vi "SigSyn (G3)-Create (1D).vi"(0 "StimChans In":T1[](array[typedef]) {"Filter"."Stages"."IIR Filter"."Forward Coefficients" format="%.4f"; "Filter"."Stages"."IIR Filter"."Reverse Coefficients" format="%.4f"}, 1 "Apply multipliers? (F)":bool, 5 "Sampling Rate (Hz)":dbl=100000.0, 7 "Npts":i32=500, 9 "Rep Num":i32=-1, 11 "error in (no error)":errorcluster, 12 "Zero unused (F)":bool) -> (4 "StimChans Out":T1[](array[typedef]) {"Filter"."Stages"."IIR Filter"."Forward Coefficients" format="%.4f"; "Filter"."Stages"."IIR Filter"."Reverse Coefficients" format="%.4f"}, 6 "Waveform":dbl[][](array[numeric]), 8 "Multipliers":dbl[](array[numeric]), 15 "error out":errorcluster)   [LabVIEW 2020]
uses:
  XControls/Stimulus Channel (G3)/Full Stimulus Channel Data.ctl
  XControls/Waveform XControls/Waveform (G3)/Waveform Data.ctl
  Waveform VIs/Waveform Enum (V3).ctl
  XControls/Waveform XControls/Tone (G3)/Tone.Properties.ctl
  Waveform VIs/Pulse Train VIs/Pulse Train Params.ctl
  Waveform VIs/Pulse Train VIs/Pulse Polarity.ctl
  Waveform VIs/Pulse Train VIs/PT-Continuous State.ctl
  Waveform VIs/Noise VIs/Noise (G3).ctl
  Waveform VIs/Noise VIs/Noise (G3).Properties.ctl
  Waveform VIs/Noise VIs/Noise (G3).Data.ctl
  Waveform VIs/File VIs/StimFile-Params.ctl
  Waveform VIs/FM Sweep VIs/FM Sweep Params.ctl
  Waveform VIs/Chirp Train VIs/Chirp Train.ctl
  Waveform VIs/Chirp Train VIs/Chirp Train Params.ctl
  Waveform VIs/Complex Tone VIs/CT-Params.ctl
  Waveform VIs/Complex Tone VIs/CT-Phase Enum.ctl
  Waveform VIs/Complex Tone VIs/CT-Runtime Data.ctl
  XControls/Waveform XControls/FM Tone/Data.ctl
  XControls/Waveform XControls/Vowel/Vowel.Properties.ctl
  Waveform VIs/Ramp VIs/Ramp.Properties.ctl
  XControls/Filter (G3)/Filter Data.ctl
  XControls/Filter (G3)/Filter Type.ctl
  Filter VIs/Filter-Bandwidth Units.ctl
  Controls/Burst XCtl/Burst Data.ctl
  XControls/Level (G3)/Level Data.ctl
  XControls/Level (G3)/Level Units (G3).ctl
  XControls/Advanced Options (G3)/Advanced Options (G3).ctl
  Modulation VIs/SAM VIs/SAM Params.ctl
  Typedefs/Destination.ctl
  PXI DAQ VIs/DAQ Engine VIs/AO Gain and Multiplier VIs/PXI Multipliers to AO Gains (1D).vi
  XControls/Filter (G3)/Filter (G3).xctl
  XControls/Level (G3)/Level (G3).xctl
  Controls/Burst XCtl/Burst Control.xctl
  XControls/Waveform XControls/Waveform (G3)/Waveform (G3).xctl
  XControls/Stimulus Channel (G3)/Stimulus Channel (G3).xctl
  XControls/Advanced Options (G3)/Advanced Options (G3).xctl
  XControls/Waveform XControls/Tone (G3)/Tone (G3).xctl
  XControls/Waveform XControls/FM Tone/FM Tone.xctl
  XControls/Waveform XControls/Vowel/Vowel.xctl
panel:
  out "Ceilings":dbl[](array[numeric])
  out "Gains":dbl[](array[numeric])
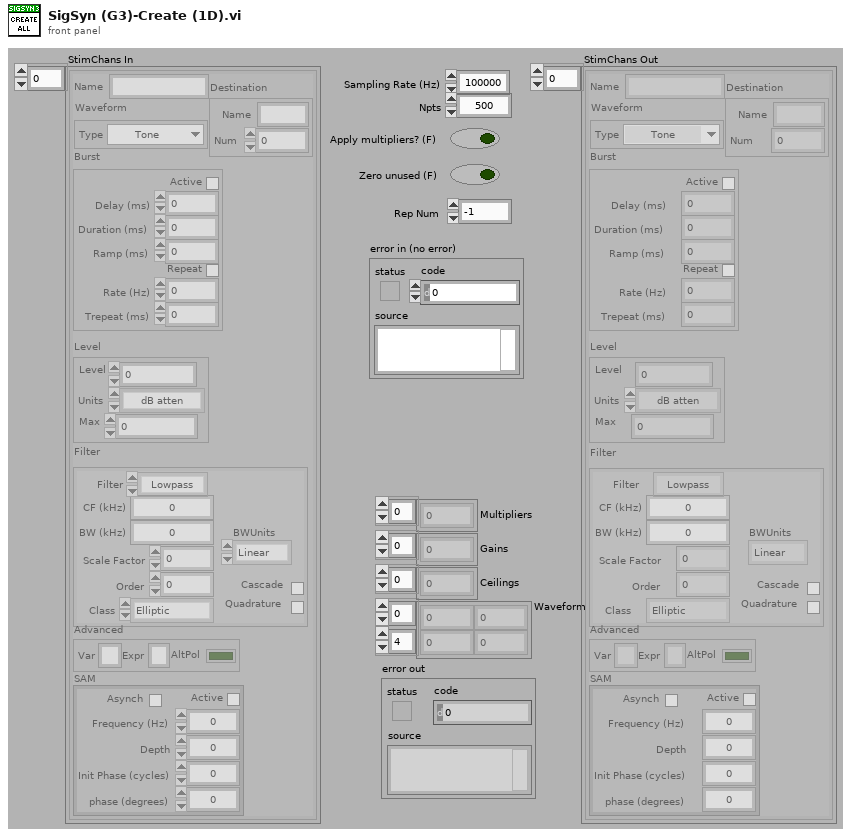
[diagram p1: front panel]
types:
  T1 = typedef "Stimulus Channel (G3).xctl/Full Stimulus Channel Data.ctl" = cluster{"Waveform":T2, "Filter":T21, "Burst":T24, "Level":T25, "Name":string, "Advanced":T27, "SAM":T28, "Destination":T29}
  T2 = typedef "Waveform (G3).xctl/Waveform Data.ctl" = cluster{"Type":T3, "Tone":T4, "Pulse Train":T5, "Noise":T8, "File":T11, "FMSweep":T12, "Chirp Train":T13, "Complex Tone":cluster{"Params":T15, "Data":T17}, "FM":T18, "Vowel":T19, "Ramp":T20}
  T3 = typedef "Waveform Enum (V3).ctl" = enum16{"OFF", "Tone", "Noise", "Pulse Train", "File", "FM Sweep", "Chirp Train", "Complex Tone", "FM Tone", "Vowel", "Ramp"}
  T4 = typedef "Tone (G3).xctl/Tone.Properties.ctl" = cluster{"Frequency (kHz)":dbl, "Phase (cycles)":dbl, "Random phase":bool}
  T5 = typedef "Pulse Train Params.ctl" = cluster{"Pulse width (us)":dbl, "Pulse rate (Hz)":dbl, "Gap (ms)":dbl, "Polarity":T6, "PT State":T7, "Asynch":bool}
  T6 = typedef "Pulse Polarity.ctl" = enum16{"POS", "NEG", "POS-NEG", "NEG-POS"}
  T7 = typedef "PT-Continuous State.ctl" = cluster{"Template":dbl[], "Nperiod":i32, "Index":i32, "Pulse Rate (Hz)":dbl, "Phase (cycles)":dbl, "Noff":i32}
  T8 = typedef "Noise (G3).ctl" = cluster{"Properties":T9, "Data":T10}
  T9 = typedef "Noise (G3).Properties.ctl" = cluster{"InvFilt":bool, "Aweight":bool, "Seed":i32, "Tokens":i32, "Brickwall":bool}
  T10 = typedef "Noise (G3).Data.ctl" = cluster{"TokenNum":i32}
  T11 = typedef "StimFile-Params.ctl" = cluster{"Filename":path, "Signal":dbl[], "Channel":i32, "stream":bool, "offset":i32, "nreps":i32, "loops":i32, "Randomize":bool, "order":i32[], "Seed":i32, "Tokens":i32}
  T12 = typedef "FM Sweep Params.ctl" = cluster{"Rate (oct/s)":dbl, "Fmin (Hz)":dbl, "Fmax (Hz)":dbl, "Ramp (ms)":dbl, "Linear":bool}
  T13 = typedef "Chirp Train.ctl" = cluster{"Params":T14, "Data":cluster{"WF":dbl[]}}
  T14 = typedef "Chirp Train Params.ctl" = cluster{"Fmin (kHz)":dbl, "Fmax (kHz)":dbl, "Compensate":bool, "Duration (ms)":dbl}
  T15 = typedef "CT-Params.ctl" = cluster{"F0 (Hz)":dbl, "Band":cluster{"Flow (Hz)":dbl, "Fhigh (Hz)":dbl}, "Phase":T16, "Min F0 (Hz)":dbl, "Max F0 (Hz)":dbl, "ContinRandPhase":bool, "Max peak factor":dbl, "Max mod depth":dbl, "MinHarmNum":i32, "MaxHarmNum":i32, "Level Mode":enum16{"per component", "overall rms"}, "% jitter":dbl}
  T16 = typedef "CT-Phase Enum.ctl" = enum16{"Cosine", "Random", "Alternating"}
  T17 = typedef "CT-Runtime Data.ctl" = cluster{"Ncomp":i32, "MinHarm":i32, "Phase":dbl[], "Amplitude":dbl[], "Npts/frame":i32, "Last F0":dbl, "Fmin":dbl, "Fmax":dbl, "Lslope":dbl, "randphase":bool, "overall rms":bool, "fmult":dbl[], "jittered":bool}
  T18 = typedef "FM Tone.xctl/Data.ctl" = cluster{"Carrier (kHz)":dbl, "ModRate (Hz)":dbl, "Depth (Hz)":dbl, "Phase (cycles)":dbl}
  T19 = typedef "Vowel.xctl/Vowel.Properties.ctl" = cluster{"Freqs":string, "Set level":enum16{"Total", "Per component"}, "Freq":dbl[], "weights":dbl[]}
  T20 = typedef "Ramp.Properties.ctl" = cluster{"Duration (ms)":dbl}
  T21 = typedef "Filter (G3).xctl/Filter Data.ctl" = cluster{"Type":T22, "CF (kHz)":dbl, "BW (kHz)":dbl, "Cascade":bool, "Quadrature":bool, "Scale Factor":dbl, "Stages":cluster{"IIR Filter":cluster{"filter structure":enum32{"IIR 2nd Order", "IIR 4th Order"}, "Reverse Coefficients":dbl[], "Forward Coefficients":dbl[]}, "State":dbl[]}[], "Class":enum16{"Elliptic", "Butterworth"}, "Order":i32, "BWUnits":T23}
  T22 = typedef "Filter (G3).xctl/Filter Type.ctl" = enum16{"OFF", "Lowpass", "Highpass", "Bandpass", "Bandstop"}
  T23 = typedef "Filter-Bandwidth Units.ctl" = enum16{"Linear", "Octaves", "Min-Max"}
  T24 = typedef "Burst Control.xctl/Burst Data.ctl" = cluster{"Active":bool, "Delay (ms)":dbl, "Duration (ms)":dbl, "Ramp (ms)":dbl, "Rate (Hz)":dbl, "Trepeat (ms)":dbl, "Repeat":bool}
  T25 = typedef "Level (G3).xctl/Level Data.ctl" = cluster{"Level":dbl, "Units":T26, "Max":dbl, "Data":cluster{"Multiplier":dbl, "Cal File":path, "Cal":cluster{"Freq (Hz)":dbl[], "Mag (dB SPL)":dbl[], "Phase (deg)":dbl[]}, "audiogram":path}}
  T26 = typedef "Level (G3).xctl/Level Units (G3).ctl" = enum16{"dB atten", "dB SPL", "dB re 1 Vrms", "dB V/Hz½", "mW", "dB HL", "Volts", "dB mW"}
  T27 = typedef "Advanced Options (G3).xctl/Advanced Options (G3).ctl" = cluster{"AltPol":bool, "Var":string, "Expr":string}
  T28 = typedef "SAM Params.ctl" = cluster{"Active":bool, "Frequency (Hz)":dbl, "Depth":dbl, "Init Phase (cycles)":dbl, "phase (degrees)":dbl, "Asynch":bool}
  T29 = typedef "Destination.ctl" = cluster{"Name":string, "Num":i32}
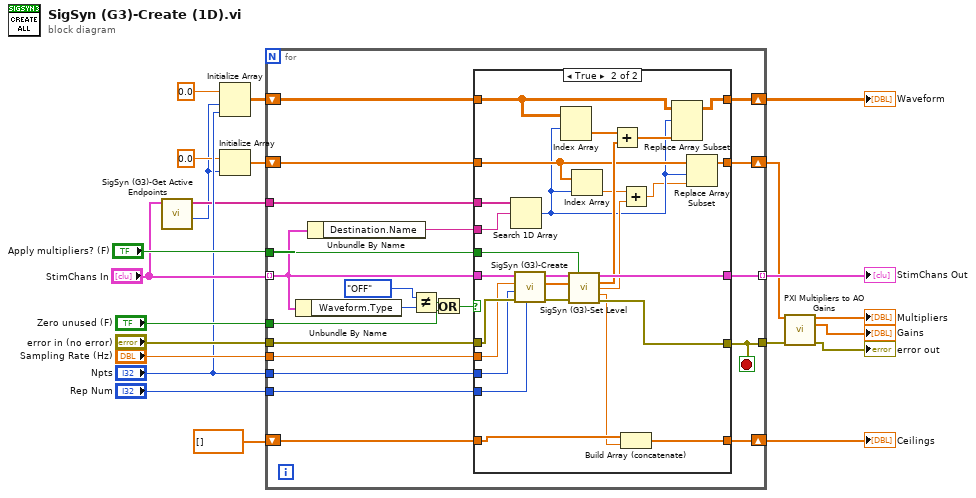
[diagram p0: block diagram]
diagram:
  n1 = call "SigSyn (G3)-Get Active Endpoints.vi"("StimChans In"="StimChans In") -> ("Num Endpoints"=w3:i32, "Active Endpoints"=w5:string[])  [unwired: 9 in]
  n2 = Initialize Array(0.0 ("Numeric"), w3, "Npts") -> (w6:dbl[][])
  n3 = Initialize Array(0.0 ("Numeric"), w3) -> (w2:dbl[])
  n4 = for {
    tunnel: [w42] -> w11 mode=indexing
    shift-right: [w40] -> w13
    shift-left: w6 -> [w41]
    shift-right: [w38] -> w17
    shift-left: dbl[] [] -> [w39]
    tunnel: "StimChans In" -> [w26] mode=indexing
    tunnel: "Sampling Rate (Hz)" -> [w37]
    tunnel: "Npts" -> [w36]
    tunnel: "Zero unused (F)" -> [w31]
    tunnel: "Apply multipliers? (F)" -> [w30]
    tunnel: "error in (no error)" -> [w43]
    tunnel: [w29] -> w10
    tunnel: "Rep Num" -> [w28]
    tunnel: w5 -> [w27]
    shift-right: [w23] -> w1
    shift-left: w2 -> [w24]
    stop <- w29 stop-if-true
    n5 = Unbundle By Name(w26) -> ("Waveform.Type"=w35:T3)
    n6 = Unbundle By Name(w26) -> ("Destination.Name"=w25:string)
    n7 = Not Equal?(x=Waveform_Enum_(V3)."OFF", y=w35) -> (x != y?=w34:bool)
    n8 = Or(x=w34, y=w31) -> (x .or. y?=w32:bool)
    n9 = case shown="True" w32 {
      tunnel: w43 -> [w47 w75]
      tunnel: [w47 w70] -> w29
      tunnel: [w45 w69] -> w42
      tunnel: w41 -> [w48 w56]
      tunnel: [w48 w55] -> w40
      tunnel: w39 -> [w46 w73]
      tunnel: [w46 w74] -> w38
      tunnel: w26 -> [w45 w65]
      tunnel: w37 -> [_ w71]
      tunnel: w36 -> [_ w72]
      tunnel: w30 -> [_ w64]
      tunnel: w28 -> [_ w63]
      tunnel: w27 -> [_ w61]
      tunnel: w25 -> [_ w60]
      tunnel: w24 -> [w44 w52]
      tunnel: [w44 w49] -> w23
      frame False {
      }
      frame True {
        n10 = Search 1D Array(1D array=w61, element=w60) -> (index of element=w51:i32)  [unwired: 1 in]
        n11 = call "SigSyn (G3)-Create.vi"("Rep Num"=w63, "error in (no error)"=w75, "Npts"=w72, "Sampling Rate (Hz)"=w71, "Stimulus Channel"=w65) -> ("error out"=w68:errorcluster, "Waveform"=w67:dbl[], "Stimulus Channel out"=w62:T1)  [unwired: 3 in, 1 out]
        n12 = Index Array(array=w56, index (row)=w51) -> (element=w59:dbl[])  [unwired: 1 in]
        n13 = call "SigSyn (G3)-Set Level.vi"("StimChans In"=w62, "Apply multiplier? (F)"=w64, "Waveform in"=w67, "error in (no error)"=w68) -> ("StimChans Out"=w69:T1, "Waveform out"=w58:dbl[], "Multiplier"=w53:dbl, "Ceiling"=w66:dbl, "error out"=w70:errorcluster)  [unwired: 7 in]
        n14 = Index Array(array=w52, index=w51) -> (element=w54:dbl)
        n15 = Add(x=w59, y=w58) -> (x+y=w57:dbl[])
        n16 = Add(x=w54, y=w53) -> (x+y=w50:dbl)
        n17 = Build Array (concatenate)(w73, w66) -> (w74:dbl[])
        n18 = Replace Array Subset(array=w56, new element=w57, index (row)=w51) -> (w55:dbl[][])  [unwired: 1 in]
        n19 = Replace Array Subset(array=w52, new element=w50, index=w51) -> (w49:dbl[])
      }
    }
  }
  "Waveform" <- w13
  "StimChans Out" <- w11
  "Ceilings" <- w17
  n20 = call-poly "PXI Multipliers to AO Gains.vi"("Multipliers in"=w1, "error in (no error)"=w10) -> ("Multipliers out"=→"Multipliers":dbl[], "Gains"=→"Gains":dbl[], "error out"=→"error out":errorcluster)  [unwired: 11 in]
